vi "FTW-TestExecutiveGUI-Core_Process.vi"(0 "FTW Actor Instance Configuration":string="{\n  \"Identity\": \"FTW Test Executive\",\n  \"InboxAddress\": \"inproc://*\",\n  \"LoggerAddress\": \"\",\n  \"Connections\": {\n    \"TestExecutive\": \"inproc://ftwTestExec\"\n  },\n  \"Publishers\": {},\n  \"Subscriptions\": {\n    \"TestExecStatusPub\": \"\"\n  },\n  \"My Data\": false,\n  \"Refresh Period\": 2\n}", 11 "ErrorIn":errorcluster) -> (15 "Error":errorcluster)   [LabVIEW 2015, in "FTW-TestExecutiveGUI-Core.lvclass"]
uses:
  FTW-TestExecutiveGUI-Core.lvclass
  FTW-TestExecutiveGUI-Core.lvclass/FTW-TestExecutiveGUI-Core.ctl
  source/actor/Instance/FTW-ActorInstance.lvclass/FTW-ActorInstance.ctl
  source/actor/JobSequencer/FTW-SEQ-Current.vi
  source/actor/Message/Base/FTW-Message.lvclass
  source/actor/Instance/FTW-ActorInstance.lvclass
  source/actor/Message/Request/FTW-Message-IncomingRequest.lvclass
  source/actor/Instance-Extended/FTW-ActorExtended.lvclass
panel:
  in  "Multicolumn Listbox 2":i32(listbox)
  out "Table Control":string[][](table)
  in  "Step":bool
  in  "Abort":bool
  in  "Pause":bool
  in  "Start":bool
  in  "Load Seq":bool
  out "Multicolumn Listbox":i32(listbox)
  # "<---- connector pane controls to the left"
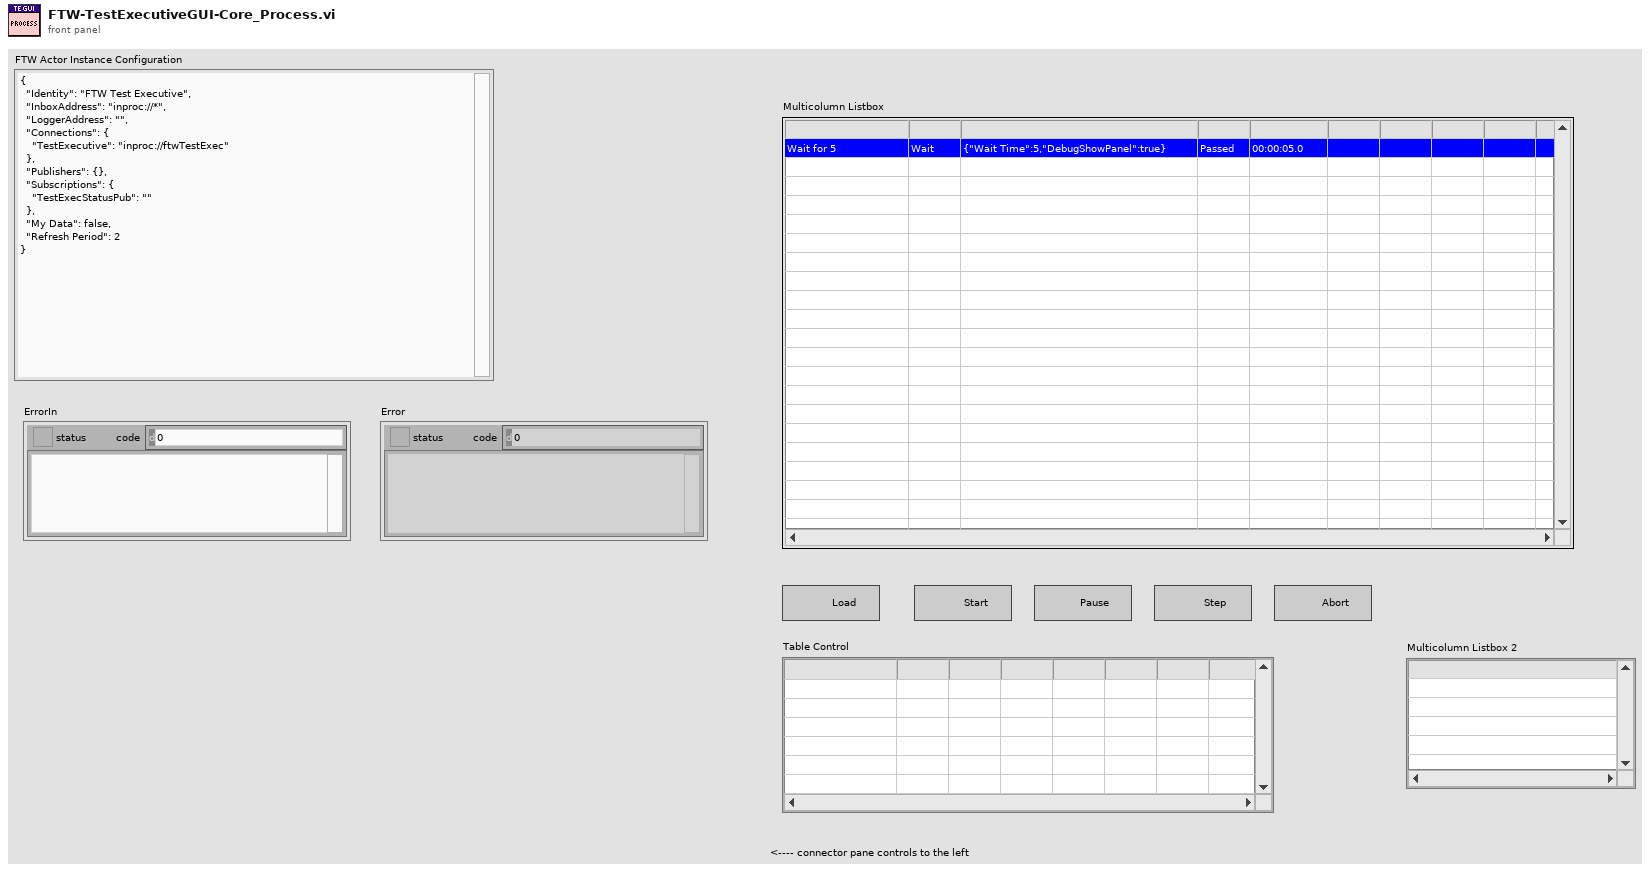
[diagram p1: front panel]
types:
  T1 = cluster{"Incoming Requests":refnum<event-registration>, "Local Messages":refnum<event-registration>, "Subscriber Registration":refnum<event-registration>}
  T2 = typedef "FTW-TestExecutive-Step.ctl" = cluster{"Name":string, "Type":string, "Path":string, "Config":string, "Elapsed Time":dbl, "Passed":bool, "State":T3, "Results":T4}
  T3 = typedef "FTW-TestExecutive-Step-State.ctl" = enum8{"None", "Failed", "Passed", "Timed out", "Aborted"}
  T4 = typedef "FTW-TestExecutive-Results.ctl" = cluster{"Start Time":timestamp, "Elapsed Time":dbl, "Passed":bool}
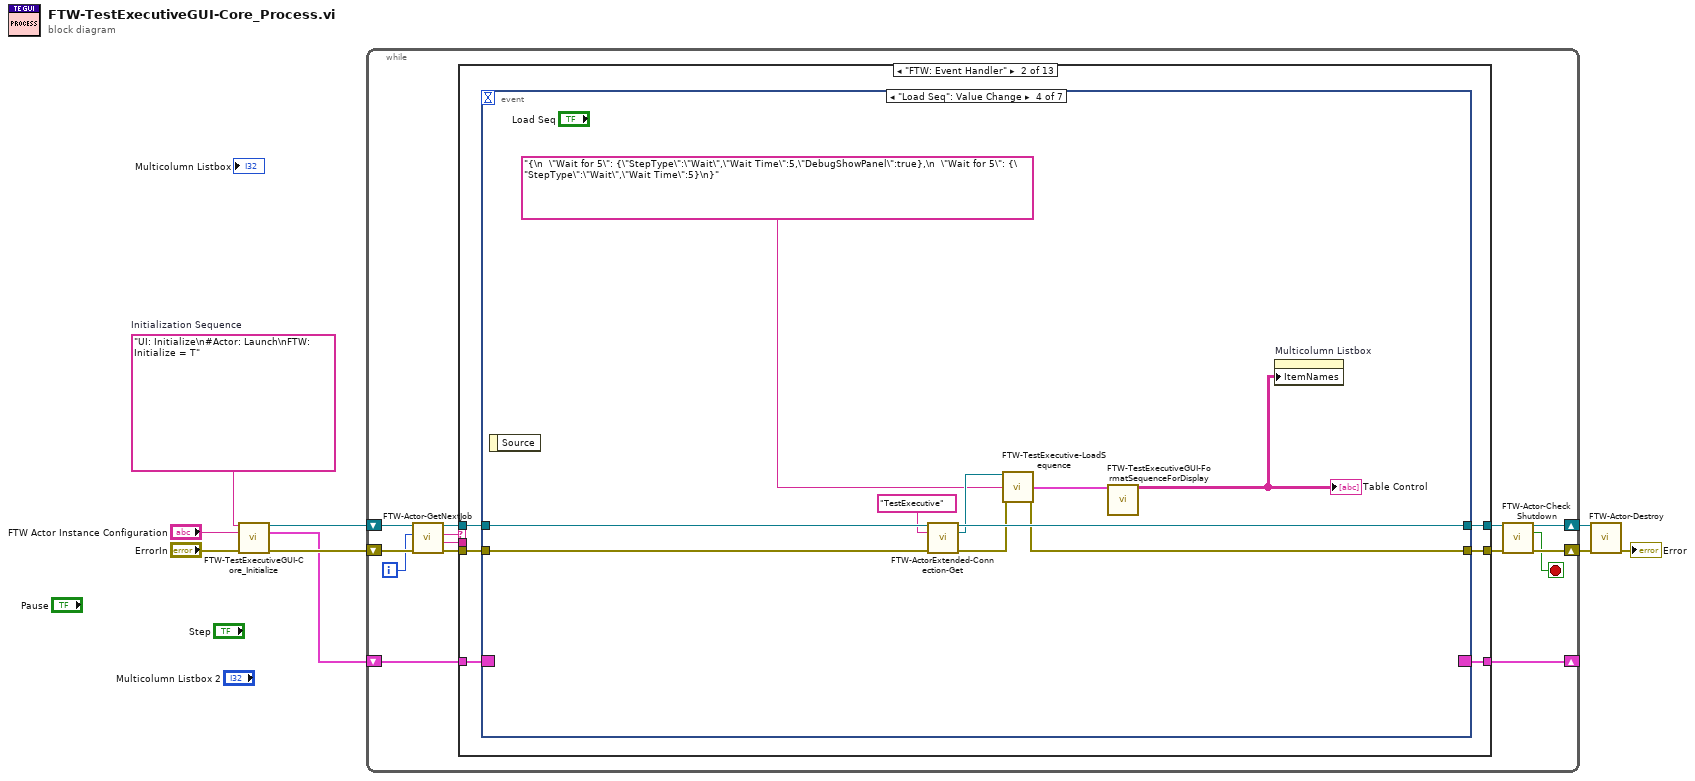
[diagram p0: block diagram]
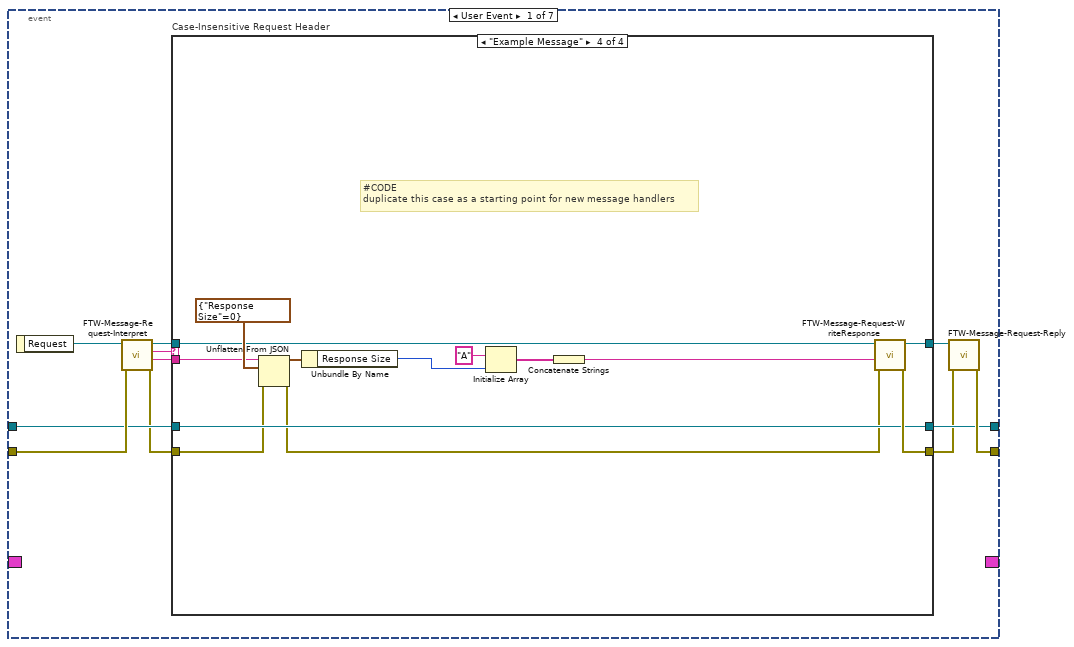
[diagram p3: hidden frame]
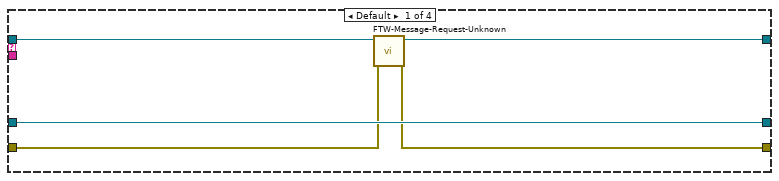
[diagram p4: hidden frame]
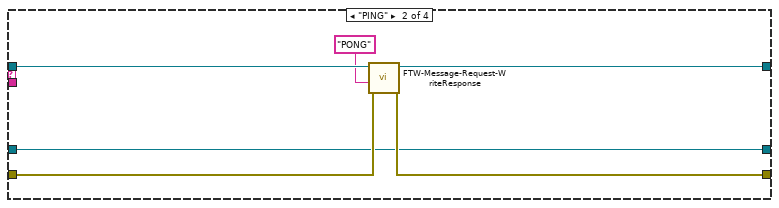
[diagram p5: hidden frame]
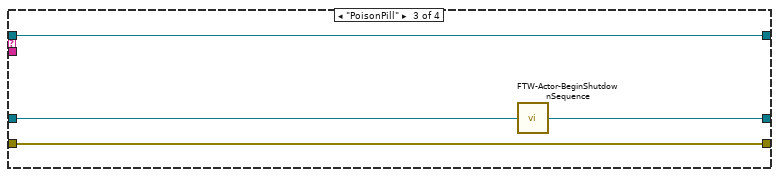
[diagram p6: hidden frame]
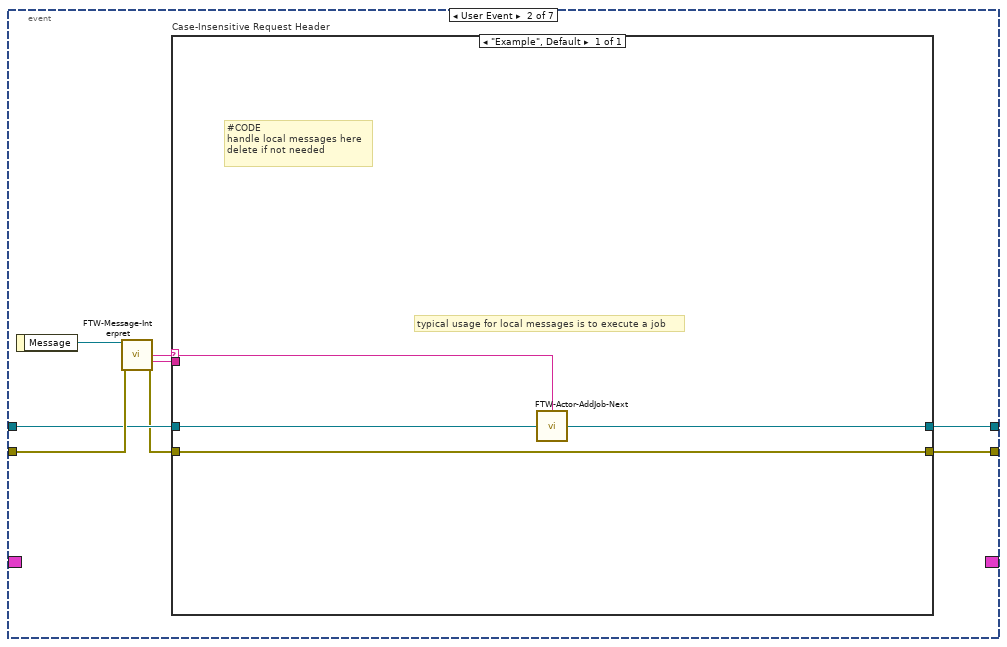
[diagram p7: hidden frame]
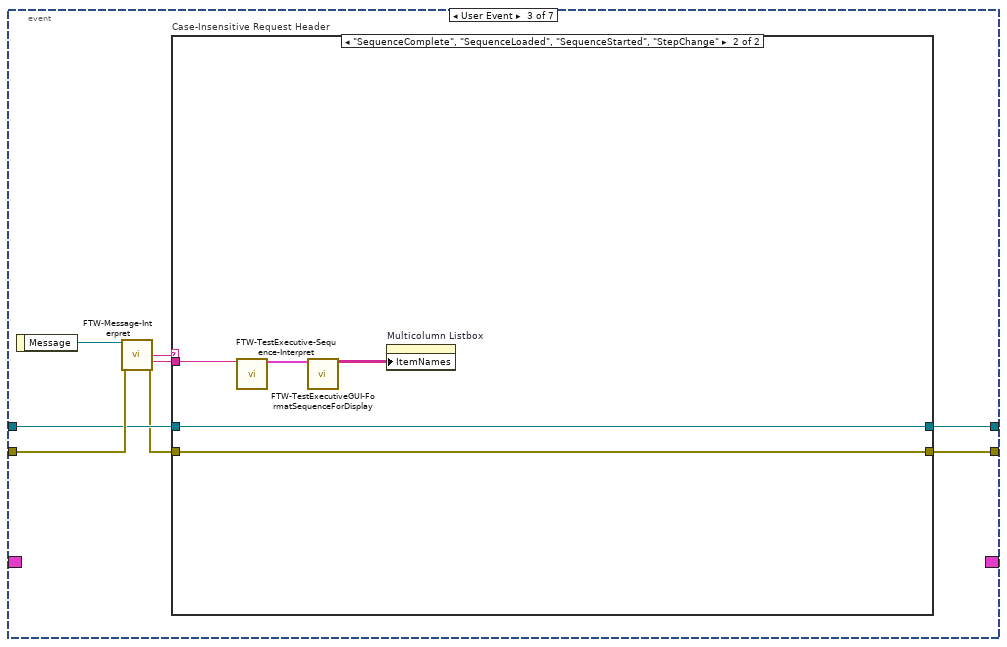
[diagram p8: hidden frame]
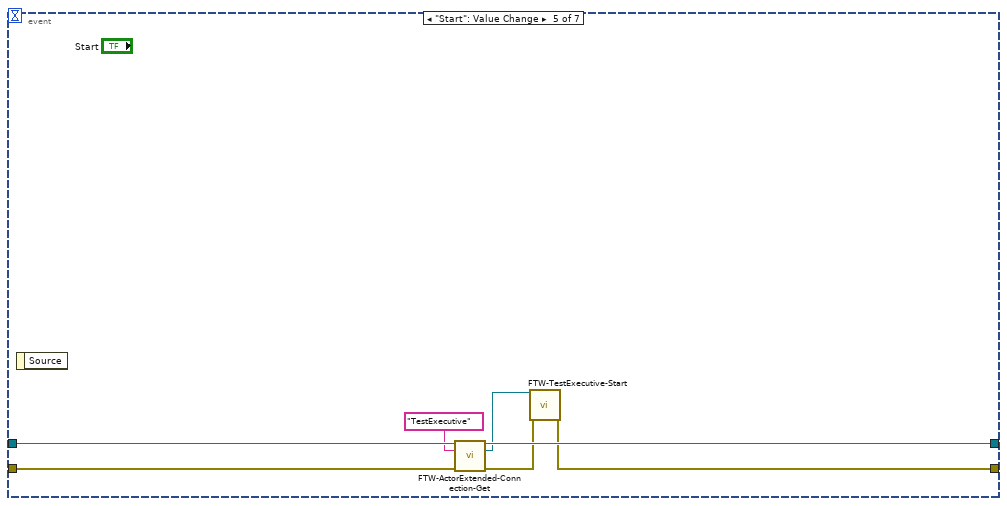
[diagram p10: hidden frame]
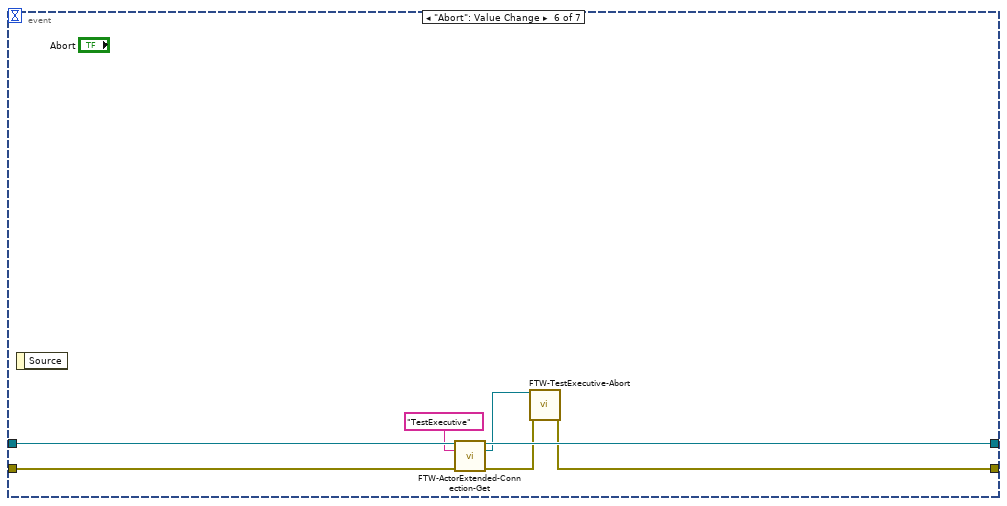
[diagram p11: hidden frame]
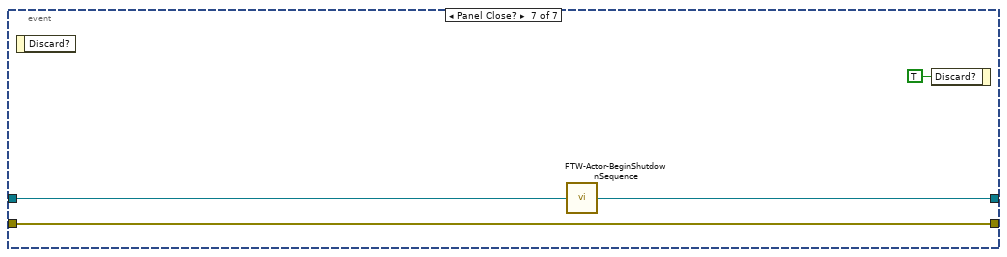
[diagram p12: hidden frame]
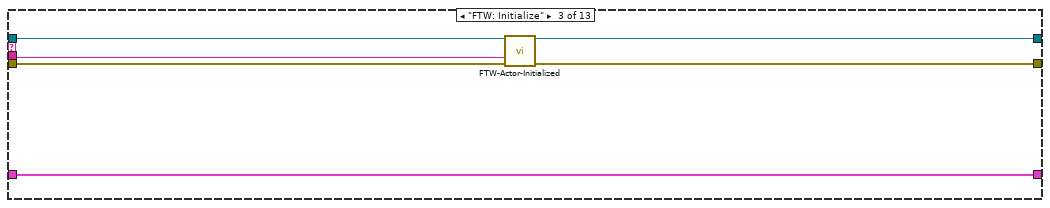
[diagram p13: hidden frame]
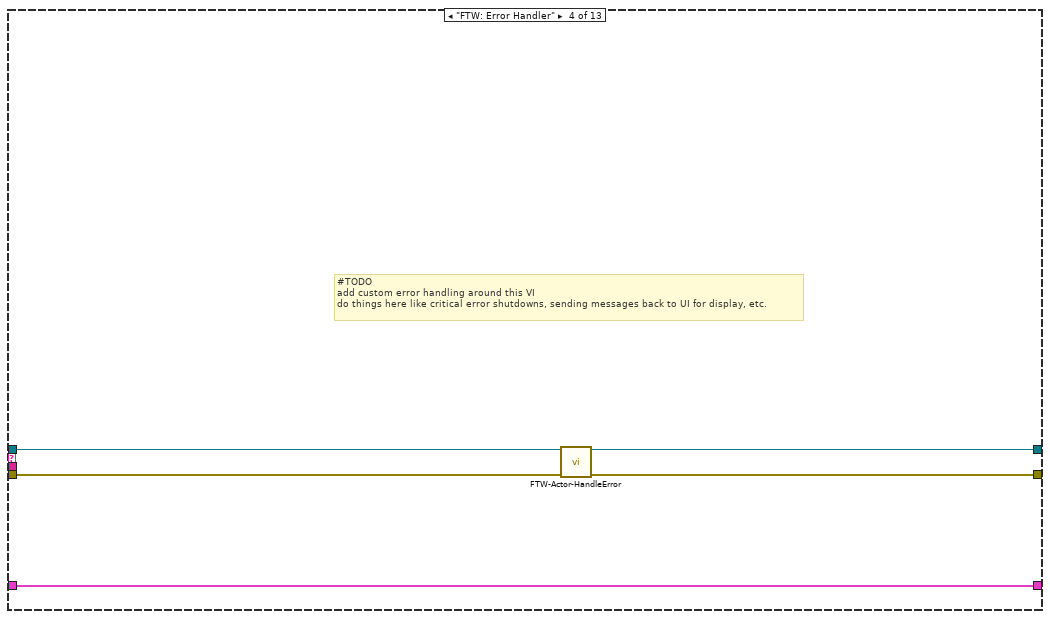
[diagram p14: hidden frame]
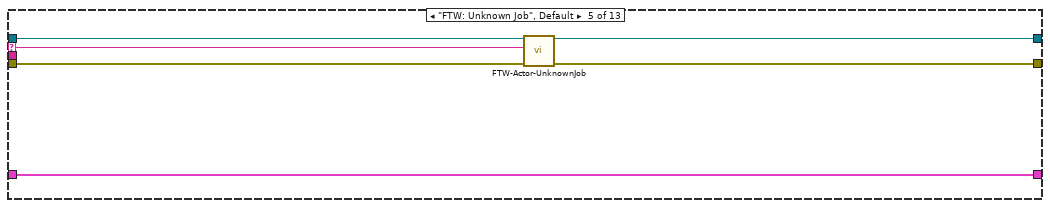
[diagram p15: hidden frame]
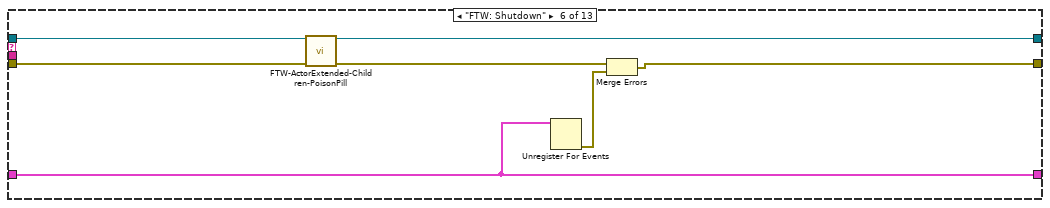
[diagram p16: hidden frame]
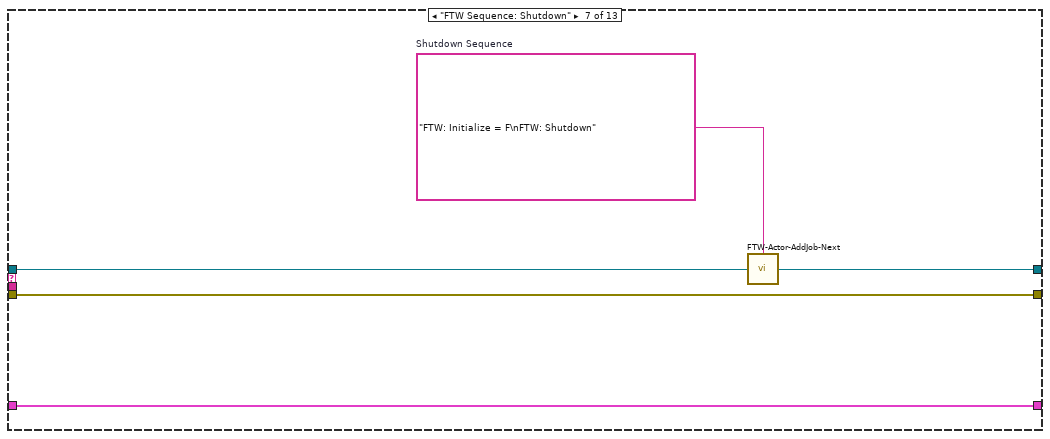
[diagram p17: hidden frame]
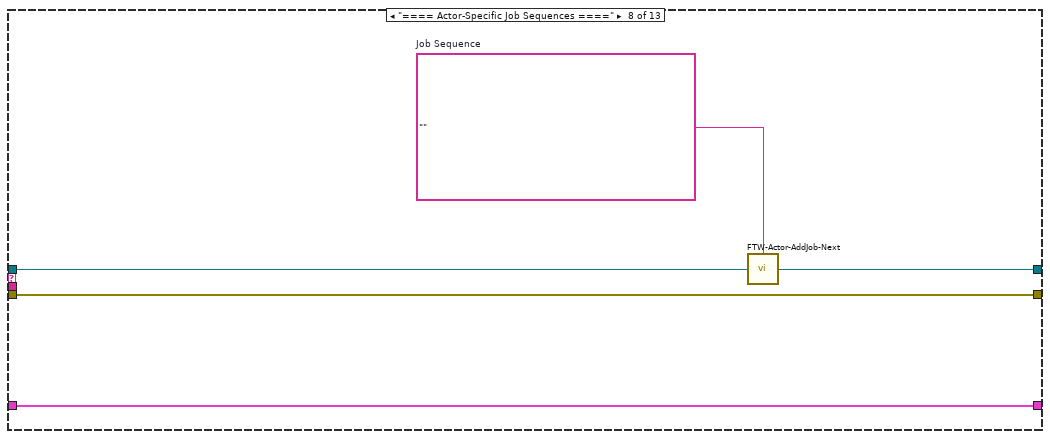
[diagram p18: hidden frame]
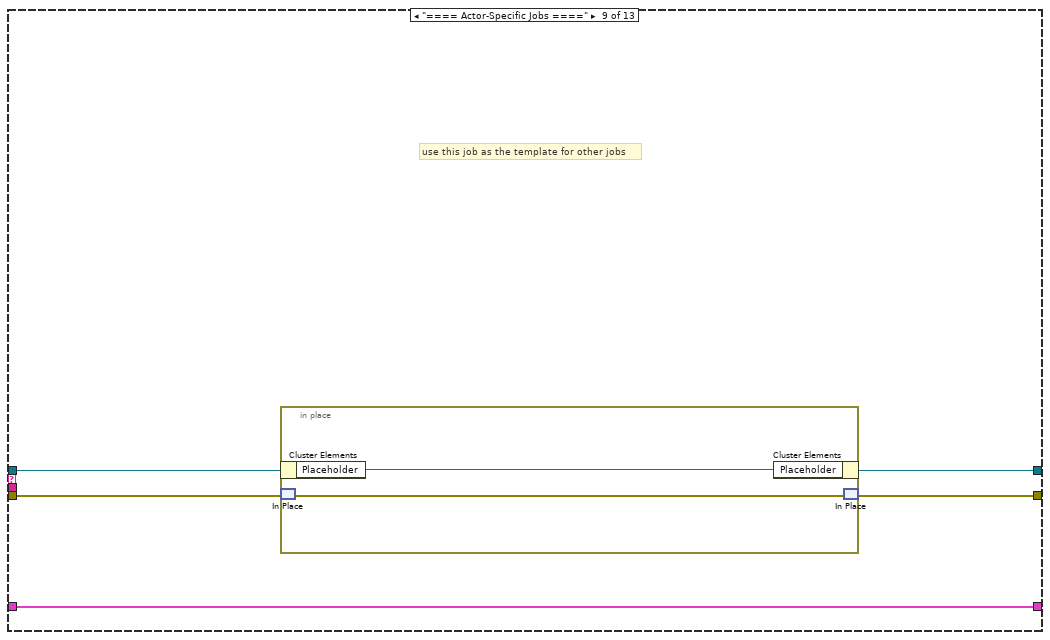
[diagram p19: hidden frame]
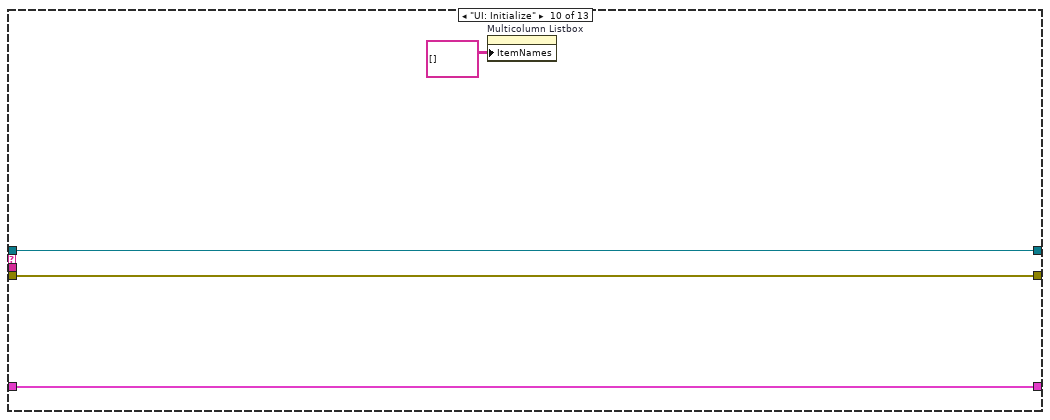
[diagram p20: hidden frame]
diagram:
  w5 = "UI: Initialize\n#Actor: Launch\nFTW: Initialize = T"  # Initialization Sequence
  n1 = call "FTW-TestExecutiveGUI-Core_Initialize.vi"("Initialization Sequence"=w5, "FTW Actor Instance Configuration"="FTW Actor Instance Configuration", "error in (no error)"="ErrorIn") -> ("Actor Template-Core out"=w2:refnum<class "FTW-TestExecutiveGUI-Core.lvclass">, "Event Refnums"=w1:T1, "error out"=w6:errorcluster)  [unwired: 9 in, 1 out]
  n2 = while {
    shift-right: [w13] -> w8
    shift-left: w6 -> [w20]
    shift-right: [w10] -> _
    shift-left: w1 -> [w23]
    shift-right: [w15] -> w9
    shift-left: w2 -> [w22]
    i -> [w11]
    stop <- w12 stop-if-true
    n3 = call "FTW-Actor-GetNextJob.vi"("error in"=w20, "Jobs Performed"=w11, "FTW Actor Instance"=w22) -> ("error out"=w19:errorcluster, "Job Data"=w17:string, "Job Name"=w18:string, "FTW Actor Instance out"=w21:refnum<class "FTW-TestExecutiveGUI-Core.lvclass">)  [unwired: 5 in]
    n4 = case shown="\"FTW: Event Handler\"" w18 {
      selector: w18 -> [_ _ _ _ w138 _ _ _ _ _ _ _ _]
      tunnel: [w25 w32 w129 w133 w141 w149 w154 w159 w163 w170 w177 w182 w188] -> w14
      tunnel: w19 -> [w25 w31 w131 w135 w142 w150 w154 w159 w164 w170 w178 w183 w194]
      tunnel: w23 -> [w26 w27 w132 w137 w143 w147 w155 w160 w165 w171 w179 w187 w195]
      tunnel: [w26 w30 w132 w137 w143 w147 w155 w160 w165 w171 w179 w187 w195] -> w10
      tunnel: w17 -> [_ _ w127 _ _ _ _ _ _ _ _ _ _]
      tunnel: [w24 w29 w130 w134 w139 w144 w152 w157 w161 w169 w175 w180 w192] -> w16
      tunnel: w21 -> [w24 w28 w128 w136 w140 w145 w153 w158 w162 w169 w176 w181 w193]
      frame "==== Featherweight Framework Jobs ====" {
      }
      frame "FTW: Event Handler" {
        n5 = event shown="[3] \"Load Seq\": Value Change" {
          selector: w27 -> [_ _ _ _ _ _ _]
          dyn-events: [_ _ _ _ _ _ _] -> w30
          timeout: _ -> [_ _ _ _ _ _ _]
          tunnel: [w42 w74 w86 w102 w109 w116 w125] -> w32
          tunnel: w31 -> [w41 w78 w90 w108 w115 w122 w125]
          tunnel: [w36 w75 w87 w106 w113 w120 w123] -> w29
          tunnel: w28 -> [w40 w77 w89 w107 w114 w121 w124]
          event User Event {
            n6 = event-data() -> ("Request"=w43:refnum<class "FTW-Message-IncomingRequest.lvclass">)  [unwired: 1 in]
            n7 = call "FTW-Message-Request-Interpret.vi"("error in"=w41, "FTW Incoming Request"=w43) -> ("error out"=w39:errorcluster, "Request Body"=w33:string, "Request Header"=w37:string, "FTW Incoming Request out"=w38:refnum<class "FTW-Message-IncomingRequest.lvclass">)  [unwired: 6 in]
            n8 = case "Case-Insensitive Request Header" shown="\"Example Message\"" w37 {
              tunnel: [w46 w52 w57 w71] -> w35
              tunnel: w39 -> [w47 w53 w57 w60]
              tunnel: [w48 w51 w58 w69] -> w36
              tunnel: w40 -> [w48 w51 w56 w69]
              tunnel: w38 -> [w45 w54 w55 w61]
              tunnel: [w44 w50 w55 w70] -> w34
              tunnel: w33 -> [_ _ _ w59]
              frame Default {
                n9 = call "FTW-Message-Request-Unknown.vi"("error in"=w47, "FTW Incoming Request"=w45) -> ("error out"=w46:errorcluster, "FTW Incoming Request Out"=w44:refnum<class "FTW-Message-IncomingRequest.lvclass">)  [unwired: 8 in]
              }
              frame "PING" {
                n10 = call "FTW-Message-Request-WriteResponse.vi"("error in"=w53, "Response Body"="PONG" ("Response Header"), "FTW Incoming Request"=w54) -> ("error out"=w52:errorcluster, "FTW Incoming Request out"=w50:refnum<class "FTW-Message-IncomingRequest.lvclass">)  [unwired: 7 in]
              }
              frame "PoisonPill" {
                n11 = call "FTW-Actor-BeginShutdownSequence.vi"("FTW Actor Instance"=w56) -> ("FTW Actor Instance out"=w58:refnum<class "FTW-TestExecutiveGUI-Core.lvclass">)  [unwired: 3 in]
              }
              frame "Example Message" {
                # "#CODE\nduplicate this case as a starting point for new message handlers"
                n12 = Unflatten From JSON(JSON string=w59, type and defaults=cluster{"Response Size":i32} {"Response Size"=0}, error in (no error)=w60) -> (value=w66:cluster{"Response Size":i32}, error out=w68:errorcluster)  [unwired: 4 in]
                n13 = Unbundle By Name(w66) -> ("Response Size"=w65:i32)
                n14 = Initialize Array("A", w65) -> (w63:string[])
                n15 = Concatenate Strings(w63) -> (w62:string)
                n16 = call "FTW-Message-Request-WriteResponse.vi"("error in"=w68, "Response Body"=w62, "FTW Incoming Request"=w61) -> ("error out"=w71:errorcluster, "FTW Incoming Request out"=w70:refnum<class "FTW-Message-IncomingRequest.lvclass">)  [unwired: 7 in]
              }
            }
            n17 = call "FTW-Message-Request-Reply.vi"("FTW: Reply Error"=w35, "FTW Incoming Request"=w34) -> ("error out"=w42:errorcluster)  [unwired: 8 in, 1 out]
          }
          event User Event {
            n18 = event-data() -> ("Message"=w79:refnum<class "FTW-Message.lvclass">)  [unwired: 1 in]
            n19 = call-dynamic "FTW-Message-Interpret.vi"("FTW Message"=w79, "error in"=w78) -> ("Message Header"=w73:string, "Message Body"=w72:string, "error out"=w76:errorcluster)  [unwired: 9 in, 2 out]
            n20 = case "Case-Insensitive Request Header" shown="\"Example\", Default" w73 {
              selector: w73 -> [w80]
              tunnel: [w82] -> w74
              tunnel: w76 -> [w82]
              tunnel: [w81] -> w75
              tunnel: w77 -> [w83]
              tunnel: w72 -> [_]
              frame "Example", Default {
                # "#CODE\nhandle local messages here\ndelete if not needed"
                # "typical usage for local messages is to execute a job"
                n21 = call "FTW-Actor-AddJob-Next.vi"("Add Next in Job Queue"=w80, "FTW Actor Instance"=w83) -> ("FTW Actor Instance out"=w81:refnum<class "FTW-TestExecutiveGUI-Core.lvclass">)  [unwired: 2 in]
              }
            }
          }
          event User Event {
            n22 = event-data() -> ("Message"=w91:refnum<class "FTW-Message.lvclass">)  [unwired: 1 in]
            n23 = call-dynamic "FTW-Message-Interpret.vi"("FTW Message"=w91, "error in"=w90) -> ("Message Header"=w85:string, "Message Body"=w84:string, "error out"=w88:errorcluster)  [unwired: 9 in, 2 out]
            n24 = case "Case-Insensitive Request Header" shown="\"SequenceComplete\", \"SequenceLoaded\", \"SequenceStarted\", \"StepChange\"" w85 {
              tunnel: [w92 w97] -> w86
              tunnel: w88 -> [w92 w97]
              tunnel: [w93 w98] -> w87
              tunnel: w89 -> [w93 w98]
              tunnel: w84 -> [_ w96]
              frame Default {
                # "#CODE\nhandle subscribed messages here if you use a subscriber\ndelete if not needed"
              }
              frame "SequenceComplete", "SequenceLoaded", "SequenceStarted", "StepChange" {
                n25 = call "FTW-TestExecutive-Sequence-Interpret.vi"("JSON"=w96) -> ("Sequence"=w94:T2[])  [unwired: 13 in, 1 out]
                n26 = call "FTW-TestExecutiveGUI-FormatSequenceForDisplay.vi"("Sequence"=w94) -> ("Table"=w95:string[][])  [unwired: 13 in, 1 out]
                n27 = property on="Multicolumn Listbox" class="MCListbox (strict)"("ItemNames"=w95) -> ()  [unwired: 2 in, 2 out]
              }
            }
          }
          event "Load Seq": Value Change {
            n28 = event-data() -> ()  [unwired: 1 in, 1 out]
            n29 = call "FTW-ActorExtended-Connection-Get.vi"("FTW-ActorExtended In"=w107, "Connector Name"="TestExecutive", "error in"=w108) -> ("FTW-ActorExtended Out"=w106:refnum<class "FTW-TestExecutiveGUI-Core.lvclass">, "FTW Actor Connector"=w104:refnum<class "FTW-ActorConnector.lvclass">, "error out"=w103:errorcluster)  [unwired: 10 in]
            n30 = call "FTW-TestExecutive-LoadSequence.vi"("FTW Actor Connector In"=w104, "Script"="{\n  \"Wait for 5\": {\"StepType\":\"Wait\",\"Wait Time\":5,\"DebugShowPanel\":true},\n  \"Wait for 5\": {\"StepType\":\"Wait\",\"Wait Time\":5}\n}", "error in (no error)"=w103) -> ("Loaded Sequence"=w100:T2[], "error out"=w102:errorcluster)  [unwired: 9 in, 2 out]
            n31 = call "FTW-TestExecutiveGUI-FormatSequenceForDisplay.vi"("Sequence"=w100) -> ("Table"=w99:string[][])  [unwired: 13 in, 1 out]
            "Table Control" <- w99
            n32 = property on="Multicolumn Listbox" class="MCListbox (strict)"("ItemNames"=w99) -> ()  [unwired: 2 in, 2 out]
          }
          event "Start": Value Change {
            n33 = event-data() -> ()  [unwired: 1 in, 1 out]
            n34 = call "FTW-ActorExtended-Connection-Get.vi"("FTW-ActorExtended In"=w114, "Connector Name"="TestExecutive", "error in"=w115) -> ("FTW-ActorExtended Out"=w113:refnum<class "FTW-TestExecutiveGUI-Core.lvclass">, "FTW Actor Connector"=w111:refnum<class "FTW-ActorConnector.lvclass">, "error out"=w110:errorcluster)  [unwired: 10 in]
            n35 = call "FTW-TestExecutive-Start.vi"("FTW Actor Connector In"=w111, "error in (no error)"=w110) -> ("error out"=w109:errorcluster)  [unwired: 10 in, 3 out]
          }
          event "Abort": Value Change {
            n36 = event-data() -> ()  [unwired: 1 in, 1 out]
            n37 = call "FTW-ActorExtended-Connection-Get.vi"("FTW-ActorExtended In"=w121, "Connector Name"="TestExecutive", "error in"=w122) -> ("FTW-ActorExtended Out"=w120:refnum<class "FTW-TestExecutiveGUI-Core.lvclass">, "FTW Actor Connector"=w118:refnum<class "FTW-ActorConnector.lvclass">, "error out"=w117:errorcluster)  [unwired: 10 in]
            n38 = call "FTW-TestExecutive-Abort.vi"("FTW Actor Connector In"=w118, "error in (no error)"=w117) -> ("error out"=w116:errorcluster)  [unwired: 10 in, 3 out]
          }
          event Panel Close? {
            n39 = event-data() -> ()  [unwired: 1 in, 1 out]
            n40 = call "FTW-Actor-BeginShutdownSequence.vi"("FTW Actor Instance"=w124) -> ("FTW Actor Instance out"=w123:refnum<class "FTW-TestExecutiveGUI-Core.lvclass">)  [unwired: 3 in]
            n41 = event-data("Discard?"=TRUE) -> ()  [unwired: 1 in, 1 out]
          }
        }
      }
      frame "FTW: Initialize" {
        n42 = call-dynamic "FTW-Actor-Initialized.vi"("FTW Actor Instance"=w128, "Positive Init?"=w127, "error in"=w131) -> ("FTW Actor Instance out"=w130:refnum<class "FTW-TestExecutiveGUI-Core.lvclass">, "error out"=w129:errorcluster)  [unwired: 11 in]
      }
      frame "FTW: Error Handler" {
        # "#TODO\nadd custom error handling around this VI\ndo things here like critical error shutdowns, sending messages back to UI for display, etc."
        n43 = call-dynamic "FTW-Actor-HandleError.vi"("FTW Actor Instance"=w136, "error in"=w135) -> ("FTW Actor Instance out"=w134:refnum<class "FTW-TestExecutiveGUI-Core.lvclass">, "error out"=w133:errorcluster)  [unwired: 10 in, 2 out]
      }
      frame "FTW: Unknown Job", Default {
        n44 = call-dynamic "FTW-Actor-UnknownJob.vi"("FTW Actor Instance"=w140, "Unknown Job"=w138, "error in"=w142) -> ("FTW Actor Instance out"=w139:refnum<class "FTW-TestExecutiveGUI-Core.lvclass">, "error out"=w141:errorcluster)  [unwired: 11 in]
      }
      frame "FTW: Shutdown" {
        n45 = call "FTW-ActorExtended-Children-PoisonPill.vi"("FTW-ActorExtended In"=w145, "error in"=w150) -> ("FTW-ActorExtended Out"=w144:refnum<class "FTW-TestExecutiveGUI-Core.lvclass">, "error out"=w146:errorcluster)  [unwired: 12 in]
        n46 = Unregister For Events(event registration refnum=w147) -> (error out=w148:errorcluster)  [unwired: 1 in]
        n47 = Merge Errors(w146, w148) -> (w149:errorcluster)
      }
      frame "FTW Sequence: Shutdown" {
        w151 = "FTW: Initialize = F\nFTW: Shutdown"  # Shutdown Sequence
        n48 = call "FTW-Actor-AddJob-Next.vi"("Add Next in Job Queue"=w151, "FTW Actor Instance"=w153) -> ("FTW Actor Instance out"=w152:refnum<class "FTW-TestExecutiveGUI-Core.lvclass">)  [unwired: 2 in]
      }
      frame "==== Actor-Specific Job Sequences ====" {
        w156 = ""  # Job Sequence
        n49 = call "FTW-Actor-AddJob-Next.vi"("Add Next in Job Queue"=w156, "FTW Actor Instance"=w158) -> ("FTW Actor Instance out"=w157:refnum<class "FTW-TestExecutiveGUI-Core.lvclass">)  [unwired: 2 in]
      }
      frame "==== Actor-Specific Jobs ====" {
        # "use this job as the template for other jobs"
        n50 = in-place {
          n51 = in-place-cluster #1(w162) -> ("Placeholder"=w166:bool)
          n52 = in-place-match #2(w164) -> (w167:errorcluster)
          n53 = in-place-cluster #1("Placeholder"=w166) -> (w161:refnum<class "FTW-TestExecutiveGUI-Core.lvclass">)
          n54 = in-place-match #2(w167) -> (w163:errorcluster)
        }
      }
      frame "UI: Initialize" {
        n55 = property on="Multicolumn Listbox" class="MCListbox (strict)"("ItemNames"=string[][] [] ("Item Names")) -> ()  [unwired: 2 in, 2 out]
      }
      frame "PUB: Publish" {
        # "#TODO\nyour published message here"
        n56 = call "FTW-ActorExtended-Publish.vi"("FTW-ActorExtended In"=w176, "Publisher Name"="<publisher name>", "Message Header"="My Header" ("Header"), "Message Body"="My Body" ("Header"), "error in"=w178) -> ("FTW-ActorExtended Out"=w175:refnum<class "FTW-TestExecutiveGUI-Core.lvclass">, "error out"=w177:errorcluster)  [unwired: 9 in]
      }
      frame "Actor: Launch" {
        w186 = 1000  # Timeout
        # "#TODO\nreplace with your actor"
        # "template for critical child actor launch"
        n57 = vi-ref "FTW-ActorTemplate.vi"() -> (w185:refnum<vi>)
        n58 = call "FTW-ActorExtended-LaunchChildActor.vi"("FTW Actor Connector Type"=w181, "Configuration"="{\n  \"Identity\": \"Replace Me\",\n  \"InboxAddress\": \"inproc://*\",\n  \"LoggerAddress\": \"\",\n  \"DebugShowPanel\": false\n}", "Actor VI Refnum"=w185, "Timeout"=w186, "error in"=w183) -> ("FTW-ActorExtended.lvclass"=w180:refnum<class "FTW-TestExecutiveGUI-Core.lvclass">, "error out"=w182:errorcluster)  [unwired: 6 in, 3 out]
      }
      frame "CONN: Ask" {
        # "example of asking a connected actor something\n\nuse the connection to call the actor API"
        n59 = call "FTW-ActorExtended-Connection-Get.vi"("FTW-ActorExtended In"=w193, "Connector Name"="ConnectionOne" ("Publisher Name"), "error in"=w194) -> ("FTW-ActorExtended Out"=w192:refnum<class "FTW-TestExecutiveGUI-Core.lvclass">, "FTW Actor Connector"=w190:refnum<class "FTW-ActorConnector.lvclass">, "error out"=w189:errorcluster)  [unwired: 10 in]
        n60 = flat-sequence {
          tunnel: w190 -> [_]
          tunnel: w189 -> [w196]
          tunnel: [w196] -> w188
          frame #0 {
          }
        }
      }
    }
    n61 = call "FTW-Actor-CheckShutdown.vi"("FTW Actor Instance"=w16, "error in"=w14) -> ("FTW Actor Instance out"=w15:refnum<class "FTW-TestExecutiveGUI-Core.lvclass">, "Shutdown?"=w12:bool, "error out"=w13:errorcluster)  [unwired: 11 in]
  }
  n62 = call-dynamic "FTW-Actor-Destroy.vi"("FTW Actor Instance"=w9, "error in"=w8) -> ("error out"=→"Error":errorcluster)  [unwired: 13 in]
